vi "Create_Exp_Envelope.vi"(11 "Cluster in":cluster{"Array":dbl[], "Amplitudes":dbl[]}) -> (3 "Cluster out":T1)   [LabVIEW 2015]
uses:
  <vilib>/Analysis/NI_AALPro.lvlib
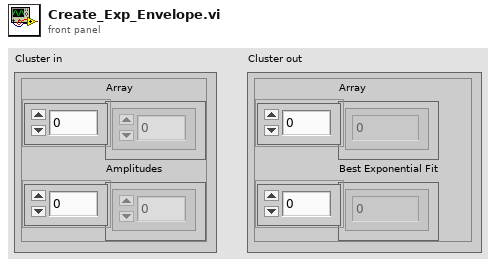
[diagram p1: front panel]
types:
  T1 = cluster{"Array":dbl[], "Best Exponential Fit":dbl[]}
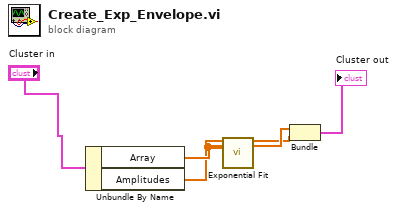
[diagram p0: block diagram]
diagram:
  n1 = Unbundle By Name("Cluster in") -> ("Array"=w5:dbl[], "Amplitudes"=w2:dbl[])
  n2 = call <vilib>:"Exponential Fit.vi"("Y"=w2, "X"=w5) -> ("Best Exponential Fit"=w3:dbl[])  [unwired: 8 in, 5 out]
  n3 = Bundle("Array"=w5, "Best Exponential Fit"=w3) -> (→"Cluster out":T1)  [unwired: 1 in]
